vi "VISA_Read_Write.vi"(7 "milliseconds to wait (50)":u32=50, 8 "error in (no error)":errorcluster, 10 "write buffer":string, 11 "VISA resource name":refnum<visa-resource-name>) -> (0 "error out":errorcluster, 1 "Transmitted String":string, 2 "read buffer":string, 3 "VISA resource name out":refnum<visa-resource-name>)   [LabVIEW 2013]
panel:
  in  "Byte Count":u32=100
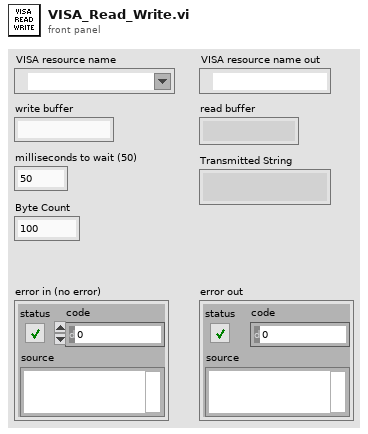
[diagram p1: front panel]
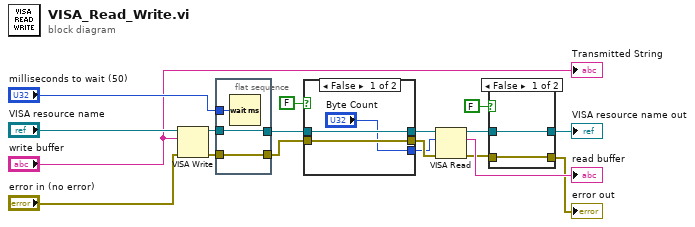
[diagram p0: block diagram]
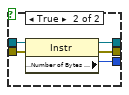
[diagram p2: hidden frame]
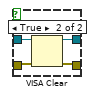
[diagram p3: hidden frame]
diagram:
  n1 = VISA Write(VISA resource name="VISA resource name", write buffer="write buffer", error in (no error)="error in (no error)") -> (VISA resource name out=w17:refnum<visa-resource-name>, error out=w18:errorcluster)  [unwired: 1 out]
  n2 = flat-sequence {
    tunnel: [w21] -> w16
    tunnel: w17 -> [w21]
    tunnel: [w20] -> w14
    tunnel: w18 -> [w20]
    tunnel: "milliseconds to wait (50)" -> [w19]
    frame #0 {
      n3 = Wait (ms)(milliseconds to wait=w19) -> ()  [unwired: 1 out]
    }
  }
  n4 = case shown="False" FALSE {
    tunnel: w16 -> [w23 w29]
    tunnel: [w23 w28] -> w15
    tunnel: w14 -> [w24 w27]
    tunnel: [w24 w26] -> w13
    tunnel: ["Byte Count" w25] -> w12
    frame False {
    }
    frame True {
      n5 = property class="Instr"(reference=w29, error in=w27) -> (reference out=w28:refnum<visa-resource-name>, error out=w26:errorcluster, "Serial Settings:Number of Bytes at Serial Port"=w25:u32)
    }
  }
  n6 = VISA Read(VISA resource name=w15, byte count=w12, error in (no error)=w13) -> (VISA resource name out=w7:refnum<visa-resource-name>, read buffer=→"read buffer":string, error out=w6:errorcluster)  [unwired: 1 out]
  n7 = case shown="False" FALSE {
    tunnel: w7 -> [w31 w35]
    tunnel: w6 -> [w30 w34]
    tunnel: [w30 w33] -> w5
    tunnel: [w31 w32] -> w4
    frame False {
    }
    frame True {
      n8 = VISA Clear(VISA resource name=w35, error in (no error)=w34) -> (VISA resource name out=w32:refnum<visa-resource-name>, error out=w33:errorcluster)
    }
  }
  "VISA resource name out" <- w4
  "error out" <- w5
  "Transmitted String" <- "write buffer"
